vi "write_T.vi"(7 "Enum":T1(ring), 8 "error in":errorcluster, 9 "Data":dbl, 10 "physical channels":tag) -> (0 "error out":errorcluster)   [LabVIEW 2015]
uses:
  <vilib>/DAQmx/write.llb/DAQmx Write (Analog DBL 1Chan 1Samp).vi
  <vilib>/DAQmx/create/channels.llb/DAQmx Create Channel (AO-Voltage-Basic).vi
  <vilib>/DAQmx/miscellaneous.llb/DAQmx Fill In Error Info.vi
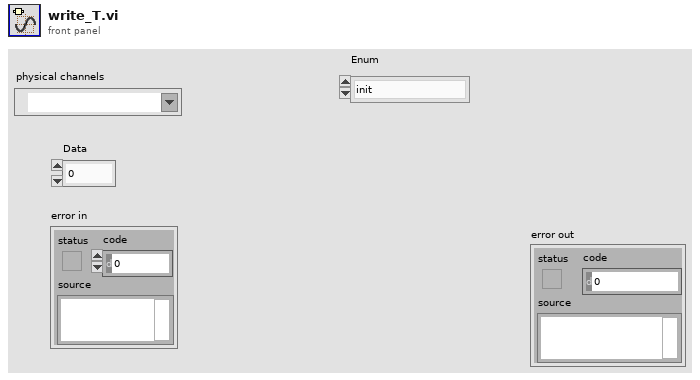
[diagram p1: front panel]
types:
  T1 = enum16{"init", "config", "start", "write", "stop"}
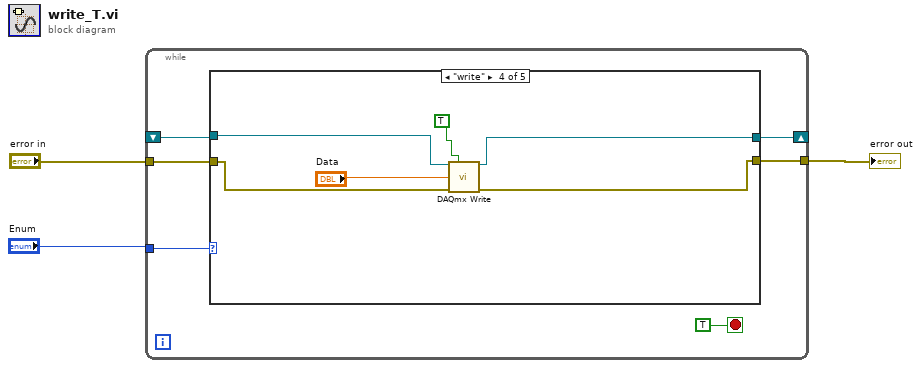
[diagram p0: block diagram]
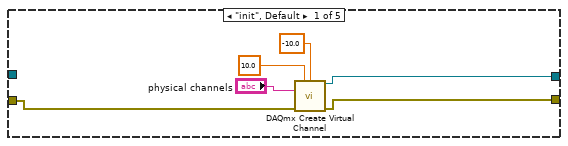
[diagram p2: hidden frame]
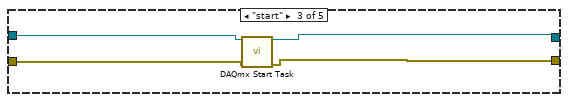
[diagram p4: hidden frame]
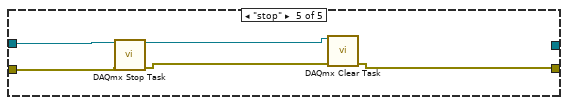
[diagram p5: hidden frame]
diagram:
  n1 = while {
    tunnel: "Enum" -> [w8]
    shift-right: [w7] -> _
    shift-left: _ -> [w6]
    tunnel: "error in" -> [w5]
    tunnel: [w4] -> w1
    stop <- TRUE stop-if-true
    n2 = case shown="\"write\"" w8 {
      tunnel: [w14 w17 w20 w25 _] -> w7
      tunnel: w6 -> [_ w17 w21 w27 w32]
      tunnel: w5 -> [w12 w16 w19 w24 w31]
      tunnel: [w15 w16 w18 w23 w30] -> w4
      frame "init", Default {
        n3 = call-poly <vilib>:"DAQmx Create Virtual Channel.vi"("maximum value"=10.0, "minimum value"=-10.0, "physical channels"="physical channels", "error in"=w12) -> ("task out"=w14:refnum<k21>, "error out"=w15:errorcluster)  [unwired: 10 in]
      }
      frame "config" {
      }
      frame "start" {
        n4 = call <vilib>:"DAQmx Start Task.vi"("task/channels in"=w21, "error in"=w19) -> ("task out"=w20:refnum<k21>, "error out"=w18:errorcluster)  [unwired: 12 in]
      }
      frame "write" {
        n5 = call-poly <vilib>:"DAQmx Write.vi"("task/channels in"=w27, "auto start"=TRUE, "data"="Data", "error in"=w24) -> ("task out"=w25:refnum<k21>, "error out"=w23:errorcluster)  [unwired: 9 in, 1 out]
      }
      frame "stop" {
        n6 = call <vilib>:"DAQmx Stop Task.vi"("task/channels in"=w32, "error in"=w31) -> ("task out"=w29:refnum<k21>, "error out"=w28:errorcluster)  [unwired: 12 in]
        n7 = call <vilib>:"DAQmx Clear Task.vi"("task in"=w29, "error in"=w28) -> ("error out"=w30:errorcluster)  [unwired: 13 in]
      }
    }
  }
  "error out" <- w1
